vi "Get Added Relays.vi"(8 "error in":errorcluster, 11 "Custom Device Ref in":T1 format="%.0x") -> (0 "error out":errorcluster, 2 "Added Relays Array":string[](array[string]), 3 "Custom Device Ref out":T1 format="%.0x")   [LabVIEW 2013, in "MUX Custom Device.lvlib"]
uses:
  MUX Custom Device.lvlib
  <vilib>/NI Veristand/Custom Device API/Custom Device Item Ref.ctl
  <vilib>/NI Veristand/Custom Device API/Custom Device API.lvlib
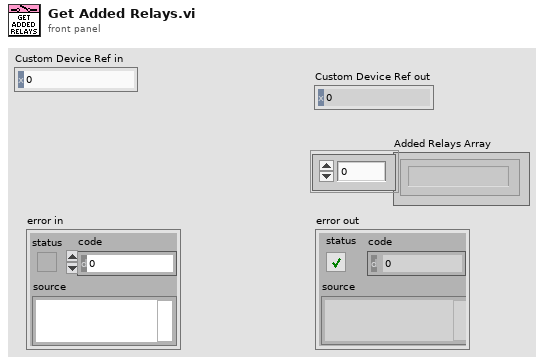
[diagram p1: front panel]
types:
  T1 = typedef "Custom Device API.lvlib/Custom Device Item Ref.ctl" = u64
  T2 = typedef "MUX Custom Device.lvlib/Relay Data.ctl" = cluster{"Relay Name":string, "State":T3}
  T3 = typedef "MUX Custom Device.lvlib/Switch.ctl" = bool
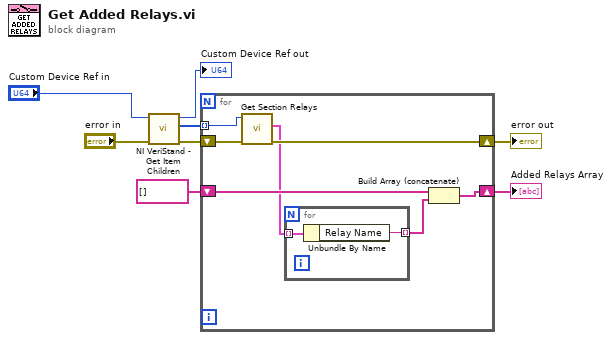
[diagram p0: block diagram]
diagram:
  n1 = call <vilib>:"NI VeriStand - Get Item Children.vi"("error in (no error)"="error in", "Item Ref in"="Custom Device Ref in") -> ("error out"=w2:errorcluster, "Child Refs"=w6:T1[], "Item Ref out"=→"Custom Device Ref out":T1)  [unwired: 6 in, 1 out]
  n2 = for {
    tunnel: w6 -> [w13] mode=indexing
    shift-right: [w11] -> w4
    shift-left: string[] [] ("Section Relays Array") -> [w12]
    shift-right: [w14] -> w8
    shift-left: w2 -> [w15]
    n3 = call "Get Section Relays.vi"("error in (no error)"=w15, "MUX Section Ref in"=w13) -> ("error out"=w14:errorcluster, "Section Relays Array"=w9:T2[])  [unwired: 7 in, 1 out]
    n4 = for {
      tunnel: w9 -> [w17] mode=indexing
      tunnel: [w16] -> w10 mode=indexing
      n5 = Unbundle By Name(w17) -> ("Relay Name"=w16:string)
    }
    n6 = Build Array (concatenate)(w12, w10) -> (w11:string[])
  }
  "Added Relays Array" <- w4
  "error out" <- w8
